vi "Make White Transparent.vi"(8 "error in (no error)":errorcluster) -> (0 "error out":errorcluster)   [LabVIEW 2014, in "Endigit.lvlib"]
doc: "Splash in Main - Set Layered Window Attributes.vi\n\nDescription:\nThis VI sets the the layered window attributes of the VI specified by the Window Name input so that the front panel background appears transparent.\n\nInputs:\nvi reference in - Reference to the VI to act upon.\n\nWindow Name (\"\") - The name of the VI to act on.\n\nFade Speed (ms per step) - Sets the fade speed (ms per step).\n\nFade Direction (Fade Out) - Specifies the fade direction (out (default) or in).\n\nTransparent FP Effect? (F) - Indicates that the VI being acted upon utilizes the transparent FP effect.\n\nerror in - Standard error cluster.\n\nOutputs:\nvi reference out - Reference to the VI to act upon.\n\nWindow Name Out - The name of the VI to act on.\n\nWindow Handle - The window handle of the VI that is acted upon.\n\nerror out - Standard error cluster.\n\nDeveloped By:\nMark Ridgley\nMark.Ridgley_LabVIEW.Developer@comcast.net"
uses:
  Endigit.lvlib
  User32.dll
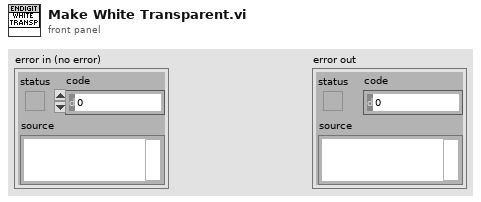
[diagram p1: front panel]
types:
  T1 = enum32{"Invalid", "Standard", "Closed", "Hidden", "Minimized", "Maximized"}
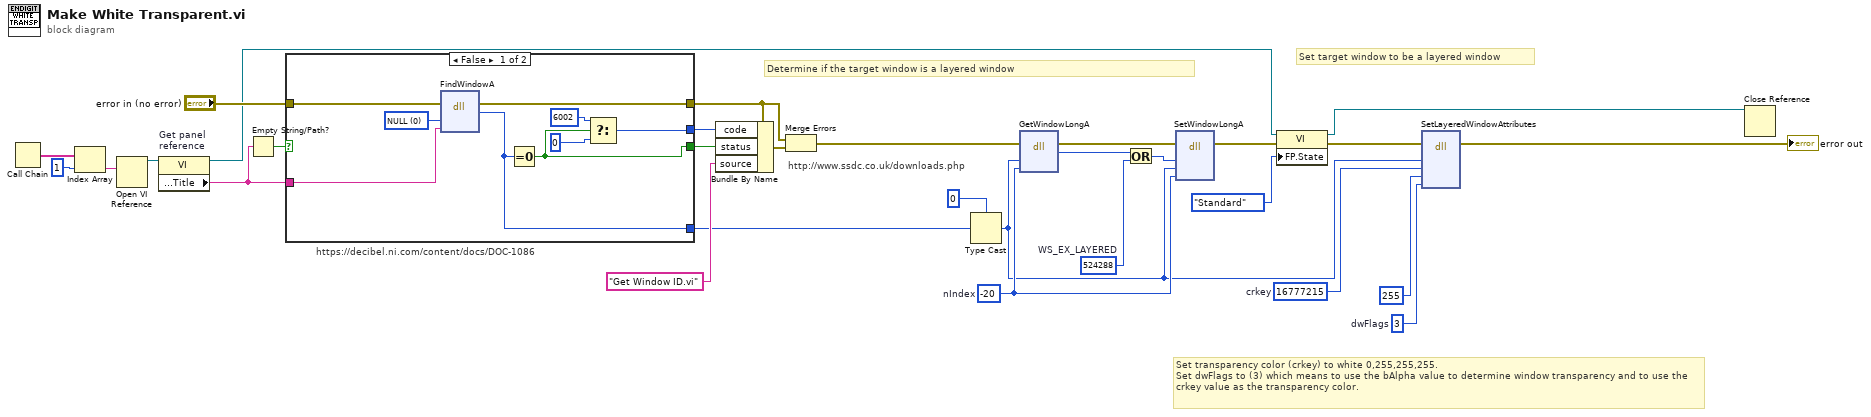
[diagram p0: block diagram]
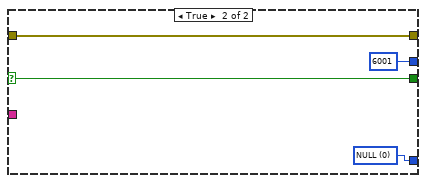
[diagram p2: hidden frame]
diagram:
  w11 = 16777215  # crkey
  w10 = 3  # dwFlags
  w14 = 524288  # WS_EX_LAYERED
  w20 = -20  # nIndex
  # "http://www.ssdc.co.uk/downloads.php"
  # "https://decibel.ni.com/content/docs/DOC-1086"
  # "Set transparency color (crkey) to white 0,255,255,255.\nSet dwFlags to (3) which means to use the bAlpha value to determine window transparency and to use the crkey value as the transparency color."
  # "Set target window to be a layered window"
  # "Determine if the target window is a layered window"
  n1 = Call Chain() -> (call chain=w28:string[])
  n2 = Index Array(array=w28, index=1) -> (element=w27:string)
  n3 = Open VI Reference(vi path=w27) -> (vi reference=w24:refnum<vi>)  [unwired: 5 in, 1 out]
  n4 = property on="Get panel\nreference" class="VI"(reference=w24) -> (reference out=w23:refnum<vi>, "Front Panel.Title"=w22:string)  [unwired: 1 in, 1 out]
  n5 = Empty String/Path?(string/path=w22) -> (empty?=w6:bool)
  n6 = case shown="False" w6 {
    selector: w6 -> [_ w41]
    tunnel: [w39 w42] -> w1
    tunnel: [w38 w41] -> w4
    tunnel: [w37 6001] -> w3
    tunnel: w22 -> [w33 _]
    tunnel: "error in (no error)" -> [w32 w40]
    tunnel: [w31 w40] -> w8
    frame False {
      w34 = 0 items=["NULL"]
      n7 = dll-call lib="user32.dll" fn="FindWindowA" label="FindWindow"(error in=w32, "lpszClassName"=w34, "lpszWindowName"=w33) -> (error out=w31:errorcluster, "hWnd"=w39:u32)  [unwired: 4 in, 1 out]
      n8 = Equal To 0?(x=w39) -> (x = 0?=w38:bool)
      n9 = Select(t=6002, s=w38, f=0) -> (s? t:f=w37:i32)
    }
    frame True {
      w42 = u16 0 items=["NULL"]
    }
  }
  n10 = Bundle By Name(cluster=w8, "code"=w3, "status"=w4, "source"="Get Window ID.vi") -> (w7:errorcluster)
  n11 = Merge Errors(w8, w7) -> (w2:errorcluster)
  n12 = Type Cast(type=0, x=w1) -> (*(type *) &x=w18:i32)
  n13 = dll-call lib="USER32.DLL" fn="GetWindowLongA" label="getWindowLong"(error in=w2, "handle"=w18, "nIndex"=w20) -> (error out=w19:errorcluster, w15:i32)  [unwired: 4 in, 1 out]
  n14 = Or(x=w15, y=w14) -> (x .or. y?=w21:i32)
  n15 = dll-call lib="USER32.DLL" fn="SetWindowLongA" label="SetWindowLong"(error in=w19, "dwNewLong"=w21, "handle"=w18, "nIndex"=w20) -> (error out=w17:errorcluster)  [unwired: 6 in, 1 out]
  n16 = property class="VI"(reference=w23, error in=w17, "FP.State"=T1."Standard" ("Front Panel Window:State")) -> (reference out=w25:refnum<vi>, error out=w12:errorcluster)
  n17 = dll-call lib="USER32.DLL" fn="SetLayeredWindowAttributes" label="SetLayeredWindowAttributs"(error in=w12, "handle"=w18, "crkey"=w11, "bAlpha"=255 ("t"), "dwFlags"=w10) -> (error out=→"error out":errorcluster)  [unwired: 7 in, 1 out]
  n18 = Close Reference(reference=w25) -> ()  [unwired: 1 in, 1 out]
